vi "Axis names.vi"(2 "Names":string[](array[string])) -> (14 "X axis name":string, 15 "Y axis name":string, 16 "Z axis name":string)   [LabVIEW 2020]
doc: "Checks if Names contains three strings for axis names. If this is not the case, it assigns X Values, Y Values and/or Z Values as the missing axis name. Sub-VI for Show_Save_Load_XY_Data.vi."
panel:
  # "This VI checks if \"Names\" contains three strings\nfor axis names. If this is not the case, it assigns\n\"X Values\", \"Y Values\" and/or \"Z Values\" as the \nmissing axis name."
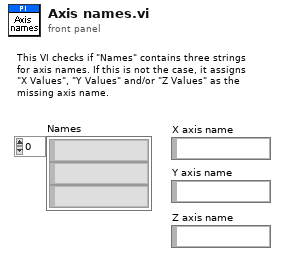
[diagram p1: front panel]
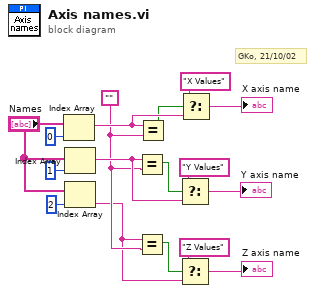
[diagram p0: block diagram]
diagram:
  w3 = ""
  # "GKo, 21/10/02"
  n1 = Index Array(array="Names", index=0 ("Index")) -> (element=w11:string)
  n2 = Index Array(array="Names", index=1 ("Index")) -> (element=w15:string)
  n3 = Index Array(array="Names", index=2 ("Index")) -> (element=w2:string)
  n4 = Equal?(x=w15, y=w3) -> (x = y?=w14:bool)
  n5 = Equal?(x=w2, y=w3) -> (x = y?=w5:bool)
  n6 = Equal?(x=w11, y=w3) -> (x = y?=w10:bool)
  n7 = Select(t="Y Values", s=w14, f=w15) -> (s? t:f=→"Y axis name":string)
  n8 = Select(t="Z Values", s=w5, f=w2) -> (s? t:f=→"Z axis name":string)
  n9 = Select(t="X Values", s=w10, f=w11) -> (s? t:f=→"X axis name":string)
